vi "Counter.vi"(1 "Reset":bool) -> (0 "Count":u8)   [LabVIEW 2019]
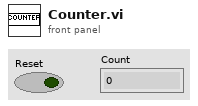
[diagram p1: front panel]
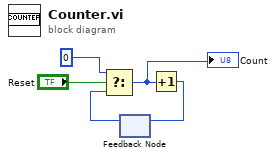
[diagram p0: block diagram]
diagram:
  n1 = feedback #1() -> (w2:u8)  [unwired: 1 in]
  n2 = Select(t=u8 0, s="Reset", f=w2) -> (s? t:f=w1:u8)
  "Count" <- w1
  n3 = Increment(x=w1) -> (x+1=w3:u8)
  n4 = feedback-in #1(w3) -> ()
